vi "Handle Tree Settings.vi"(6 "Table Setting Name in":string, 7 "Write? (F:Read)":bool, 8 "error in (no error)":errorcluster, 9 "Table Ref":refnum<vi>, 11 "Save Restore Settings in":refnum<class "Save Restore Settings.lvclass">) -> (0 "error out":errorcluster, 1 "Sub Controls":T1[](array[typedef]), 3 "Save Restore Settings out":refnum<class "Save Restore Settings.lvclass">)   [LabVIEW 2016, in "Save Restore Settings.lvclass"]
uses:
  <userlib>/_MGI/Application Control/MGI Save Restore Settings/Save Restore Settings.lvclass
  <userlib>/_MGI/Application Control/MGI Save Restore Settings/Control Info.ctl
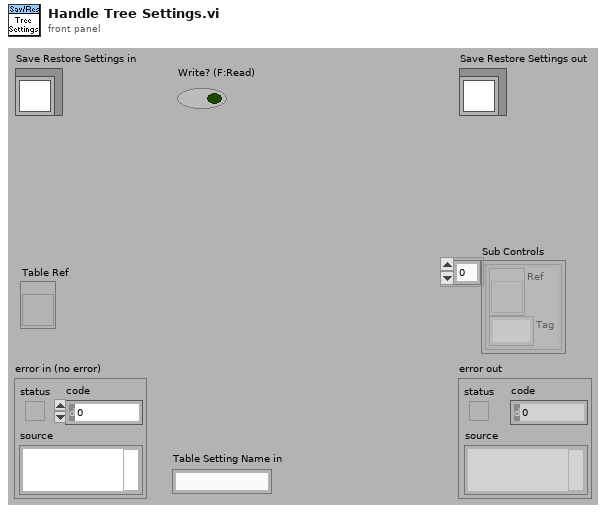
[diagram p1: front panel]
types:
  T1 = typedef "Save Restore Settings.lvclass/Control Info.ctl" = cluster{"Ref":refnum<vi>, "Tag":string}
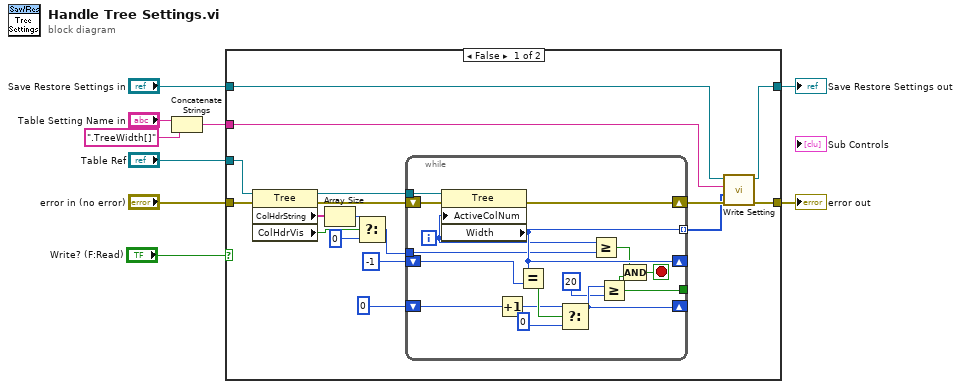
[diagram p0: block diagram]
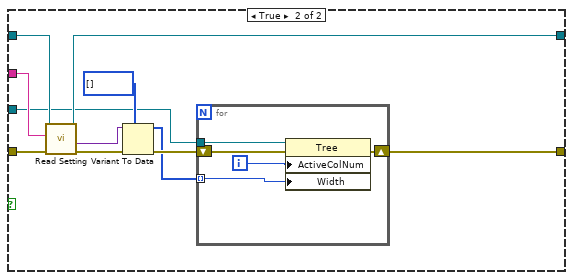
[diagram p2: hidden frame]
diagram:
  n1 = Concatenate Strings("Table Setting Name in", ".TreeWidth[]" ("string")) -> (w2:string)
  n2 = case shown="False" "Write? (F:Read)" {
    tunnel: "Table Ref" -> [w18 w45]
    tunnel: "error in (no error)" -> [w16 w51]
    tunnel: "Save Restore Settings in" -> [w26 w49]
    tunnel: [w25 w48] -> w6
    tunnel: [w24 w46] -> w5
    tunnel: w2 -> [w23 w50]
    frame False {
      n3 = property class="Tree"(reference=w18, error in=w16) -> (reference out=w17:refnum<vi>, error out=w15:errorcluster, "ColHdrString"=w13:string[], "ColHdrVis"=w14:bool)
      n4 = Array Size(array=w13) -> (size(s)=w12:i32)
      n5 = Select(t=w12, s=w14, f=0) -> (s? t:f=w10:i32)
      n6 = while {
        shift-right: [w30] -> w22
        shift-left: w15 -> [w41]
        tunnel: w17 -> [w42]
        shift-right: [w31] -> _
        shift-left: -1 -> [w40]
        shift-right: [w34] -> _
        shift-left: 0 -> [w38]
        tunnel: [w32] -> _
        tunnel: [w31] -> w19 mode=indexing
        tunnel: w10 -> [w27]
        i -> [w29]
        stop <- w35 stop-if-true
        n7 = property class="Tree"(reference=w42, error in=w41, "ActiveColNum"=w29) -> (error out=w30:errorcluster, "Width"=w31:i32)  [unwired: 1 out]
        n8 = Increment(x=w38) -> (x+1=w37:i32)
        n9 = Equal?(x=w31, y=w40) -> (x = y?=w39:bool)
        n10 = Select(t=w37, s=w39, f=0) -> (s? t:f=w34:i32)
        n11 = Greater Or Equal?(x=w29, y=w27) -> (x >= y?=w28:bool)
        n12 = Greater Or Equal?(x=w34, y=20) -> (x >= y?=w32:bool)
        n13 = Compound Arithmetic op=AND(w28, w32) -> (w35:bool)
      }
      n14 = call-dynamic "Write Setting.vi"("error in (no error)"=w22, "Tag Attribute"=w19, "Tag Name"=w23, "Save Restore Settings in"=w26) -> ("error out"=w24:errorcluster, "Save Restore Settings out"=w25:refnum<class "Save Restore Settings.lvclass">)  [unwired: 6 in]
    }
    frame True {
      n15 = call-dynamic "Read Setting.vi"("error in (no error)"=w51, "Tag Name"=w50, "Save Restore Settings in"=w49) -> ("error out"=w52:errorcluster, "Tag Attribute"=w53:variant, "Save Restore Settings out"=w48:refnum<class "Save Restore Settings.lvclass">)  [unwired: 6 in]
      n16 = Variant To Data(error in=w52, type=i32[] [], Variant=w53) -> (data=w43:i32[], error out=w44:errorcluster)
      n17 = for {
        shift-right: [w57] -> w46
        shift-left: w44 -> [w55]
        tunnel: w45 -> [w58]
        tunnel: w43 -> [w56] mode=indexing
        i -> [w54]
        n18 = property class="Tree"(reference=w58, error in=w55, "ActiveColNum"=w54, "Width"=w56) -> (error out=w57:errorcluster)  [unwired: 1 out]
      }
    }
  }
  "error out" <- w5
  "Save Restore Settings out" <- w6
